vi "get channels mapped to tag.vi"(8 "error in":errorcluster, 10 "tag":refnum<class "tag descriptor.lvclass">, 11 "engine configuration in":refnum<class "engine configuration.lvclass">) -> (0 "error out":errorcluster, 1 "readers":T1[](array[typedef]), 2 "writer":T1, 3 "engine configuration out":refnum<class "engine configuration.lvclass">)   [LabVIEW 2013, in "engine configuration.lvclass"]
uses:
  engine configuration.lvclass
  <vilib>/NI/Tag Bus/tag/tag descriptor.lvclass
  unique channel identifier.ctl
  <vilib>/NI/Tag Bus/tag/tag descriptor.lvclass/tag descriptor.ctl
  engine configuration.lvclass/engine configuration.ctl
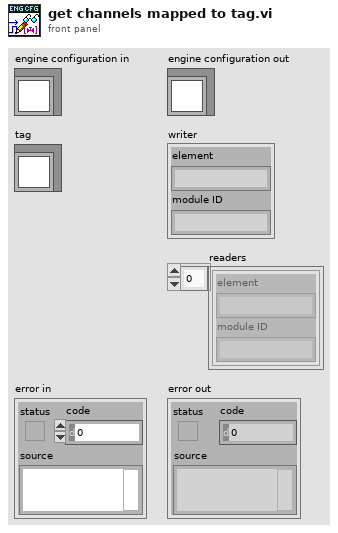
[diagram p1: front panel]
types:
  T1 = typedef "engine configuration.lvclass/unique channel identifier.ctl" = cluster{"element":string, "module ID":string}
  T2 = typedef "engine configuration.lvclass/module channel pairings.ctl" = cluster{"modules":string[], "element":string[]}
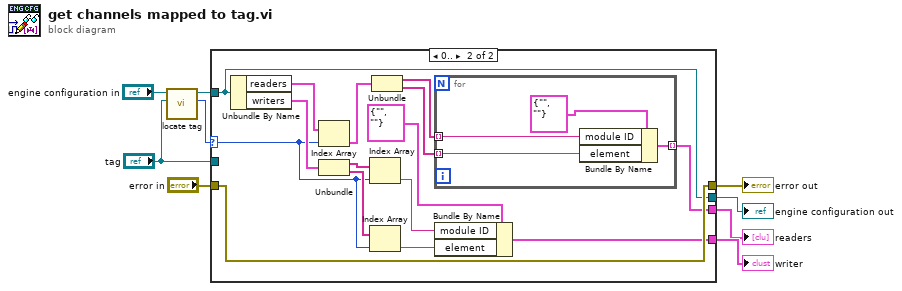
[diagram p0: block diagram]
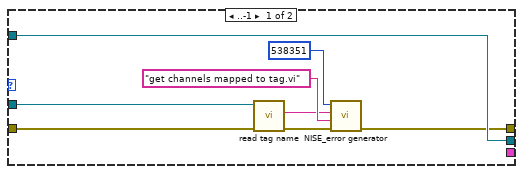
[diagram p2: hidden frame]
diagram:
  n1 = call "locate tag.vi"("tag descriptor"="tag", "engine configuration in"="engine configuration in") -> ("index"=w8:i32, "engine configuration out"=w5:refnum<class "engine configuration.lvclass">)  [unwired: 8 in]
  n2 = case shown="0.." w8 {
    selector: w8 -> [_ w26]
    tunnel: [w16 w32] -> w7
    tunnel: "error in" -> [w11 w32]
    tunnel: w5 -> [w17 w31]
    tunnel: [w17 w31] -> w4
    tunnel: "tag" -> [w13 _]
    tunnel: [_ w19] -> w2
    tunnel: [_ w18] -> w1
    frame ..-1 {
      n3 = call <vilib>:"read tag name.vi"("error in"=w11, "system tag in"=w13) -> ("error out"=w10:errorcluster, "name"=w12:string)  [unwired: 7 in, 1 out]
      n4 = call <vilib>:"NISE_error generator.vi"("error in"=w10, "source"="get channels mapped to tag.vi", "append error message"=w12, "error code (0)"=538351) -> ("error out"=w16:errorcluster)  [unwired: 5 in]
    }
    frame 0.. {
      n5 = Unbundle By Name(w31) -> ("readers"=w30:T2[], "writers"=w29:T2)
      n6 = Index Array(array=w30, index=w26) -> (element=w24:T2)
      n7 = Unbundle(w29) -> ("modules"=w28:string[], "element"=w27:string[])
      n8 = Index Array(array=w28, index=w26) -> (element=w21:string)
      n9 = Index Array(array=w27, index=w26) -> (element=w20:string)
      n10 = Unbundle(w24) -> ("modules"=w23:string[], "element"=w22:string[])
      n11 = for {
        tunnel: w23 -> [w34] mode=indexing
        tunnel: w22 -> [w35] mode=indexing
        tunnel: [w33] -> w18 mode=indexing
        n12 = Bundle By Name(cluster=T1 {"element"="", "module ID"=""} ("unique channel identifier"), "module ID"=w34, "element"=w35) -> (w33:T1)
      }
      n13 = Bundle By Name(cluster=T1 {"element"="", "module ID"=""} ("unique channel identifier"), "module ID"=w21, "element"=w20) -> (w19:T1)
    }
  }
  "error out" <- w7
  "engine configuration out" <- w4
  "writer" <- w2
  "readers" <- w1
